vi "Arm Angle Selection.vi"(9 "Vision Distance Angle":dbl, 10 "Numeric Control":u32, 11 "Shooter Data":T1) -> (2 "D4 Angle":bool, 3 "Arm Setpoint":dbl)   [LabVIEW 2015]
uses:
  <vilib>/Rock Robotics/Network Tables/NT Read Number.vi
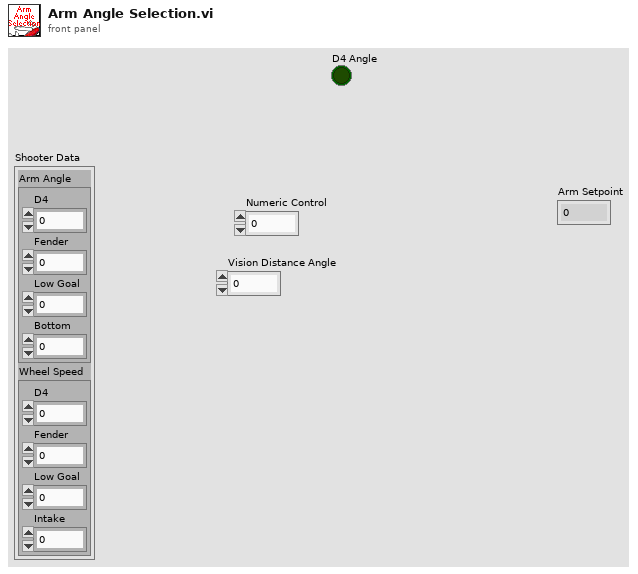
[diagram p1: front panel]
types:
  T1 = cluster{"Arm Angle":cluster{"D4":dbl, "Fender":dbl, "Low Goal":dbl, "Bottom":dbl}, "Wheel Speed":cluster{"D4":dbl, "Fender":dbl, "Low Goal":dbl, "Intake":dbl}}
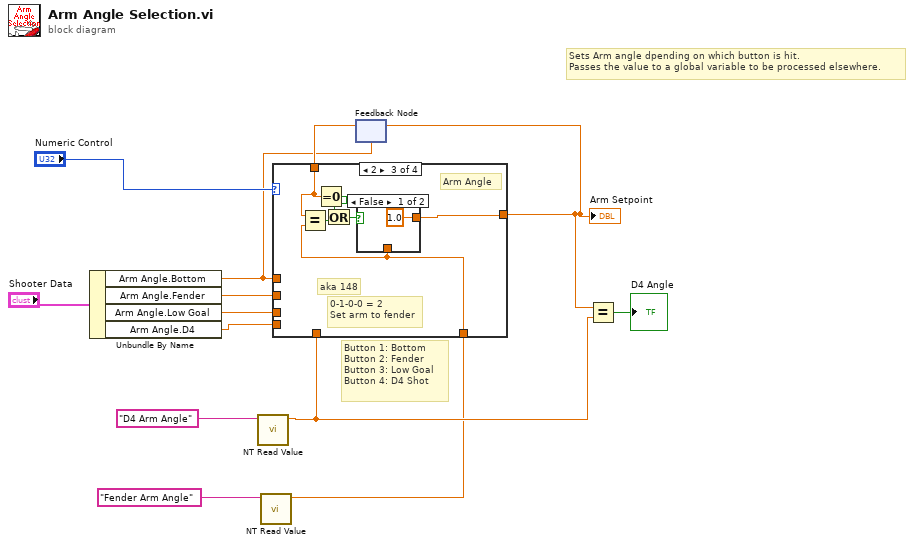
[diagram p0: block diagram]
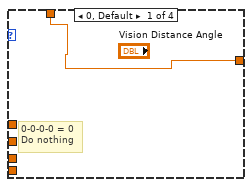
[diagram p2: hidden frame]
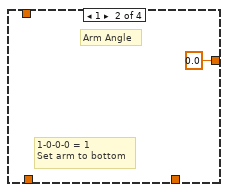
[diagram p3: hidden frame]
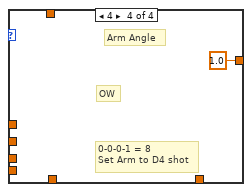
[diagram p5: hidden frame]
diagram:
  # "Button 1: Bottom\nButton 2: Fender \nButton 3: Low Goal \nButton 4: D4 Shot"
  # "Sets Arm angle dpending on which button is hit.\nPasses the value to a global variable to be processed elsewhere."
  n1 = Unbundle By Name("Shooter Data") -> ("Arm Angle.Bottom"=w10:dbl, "Arm Angle.Fender"=w9:dbl, "Arm Angle.Low Goal"=w8:dbl, "Arm Angle.D4"=w7:dbl)
  n2 = call-poly <vilib>:"NT Read Value.vi"("Name"="D4 Arm Angle") -> ("Numeric"=w4:dbl)  [unwired: 9 in, 1 out]
  n3 = call-poly <vilib>:"NT Read Value.vi"("Name"="Fender Arm Angle") -> ("Numeric"=w1:dbl)  [unwired: 9 in, 1 out]
  n4 = feedback #1(w10) -> (w13:dbl)
  n5 = case shown="2" "Numeric Control" {
    tunnel: [w14 0.0 ("Numeric") w21 1.0 ("Numeric")] -> w5
    tunnel: w13 -> [w14 _ w17 _]
    tunnel: w10 -> [_ _ _ _]
    tunnel: w9 -> [_ _ _ _]
    tunnel: w8 -> [_ _ _ _]
    tunnel: w7 -> [_ _ _ _]
    tunnel: w4 -> [_ _ _ _]
    tunnel: w1 -> [_ _ w16 _]
    frame 0, Default {
      # "0-0-0-0 = 0\nDo nothing"
    }
    frame 1 {
      # "1-0-0-0 = 1\nSet arm to bottom"
      # "Arm Angle"
    }
    frame 2 {
      # "aka 148"
      # "0-1-0-0 = 2\nSet arm to fender"
      # "Arm Angle"
      n6 = Equal?(x=w17, y=w16) -> (x = y?=w18:bool)
      n7 = Equal To 0?(x=w17) -> (x = 0?=w20:bool)
      n8 = Or(x=w20, y=w18) -> (x .or. y?=w19:bool)
      n9 = case shown="False" w19 {
        tunnel: [1.0 ("Numeric") w23] -> w21
        tunnel: w16 -> [_ w23]
        frame False {
        }
        frame True {
        }
      }
    }
    frame 4 {
      # "OW"
      # "0-0-0-1 = 8\nSet Arm to D4 shot"
      # "Arm Angle"
    }
  }
  "Arm Setpoint" <- w5
  n10 = feedback-in #1(w5) -> ()
  n11 = Equal?(x=w5, y=w4) -> (x = y?=→"D4 Angle":bool)
